vi "Select ROI Statistics Dialog.vi"(8 "error in (no error)":errorcluster) -> (0 "error out":errorcluster, 1 "OK?":bool caption="OK", 3 "ROI Statistics out":T1)   [LabVIEW 2021, in "Image.lvlib"]
doc: "Asks the user to select which ROI characteristics needs to be computed."
uses:
  Image.lvlib
  Image ROI Statistics Selection.ctl
panel:
  in  "ROI Statistics":T1
  in  "Deselect All":bool
  in  "Select All":bool
  in  "Cancel":bool
  in  "OK":bool caption="OK2"
  # "Select ROI Characteristics:"
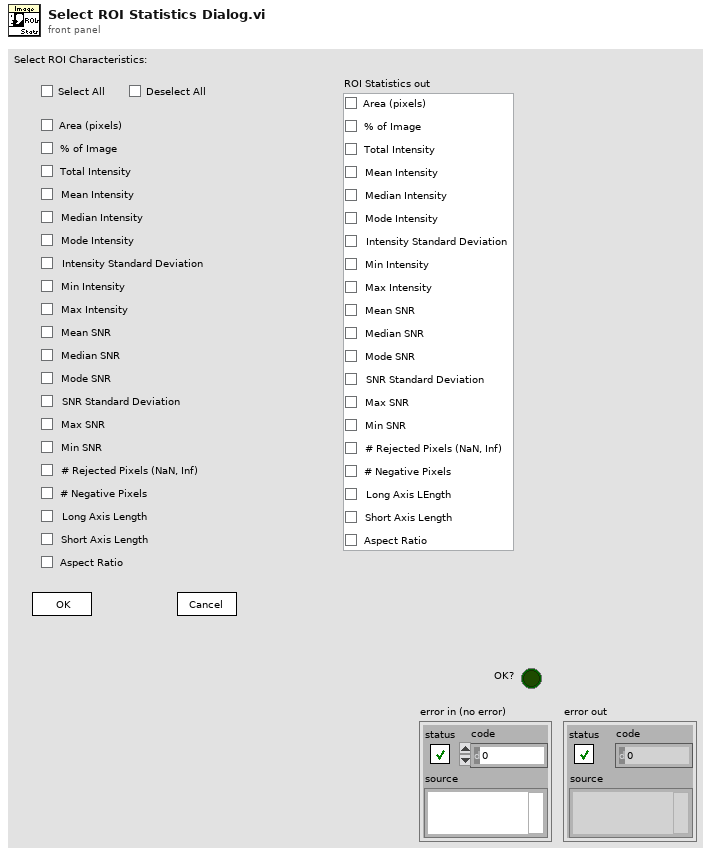
[diagram p1: front panel]
types:
  T1 = typedef "Image.lvlib/Image ROI Statistics Selection.ctl" = cluster{"Area (pixels)":bool, "% of Image":bool, "Total Intensity":bool, "Mean Intensity":bool, "Median Intensity":bool, "Mode Intensity":bool, "Intensity Standard Deviation":bool, "Min Intensity":bool, "Max Intensity":bool, "Mean SNR":bool, "Median SNR":bool, "Mode SNR":bool, "SNR Standard Deviation":bool, "Max SNR":bool, "Min SNR":bool, "# Rejected Pixels (NaN, Inf)":bool, "# Negative Pixels":bool, "Long Axis Length":bool, "Short Axis Length":bool, "Aspect Ratio":bool}
  T2 = enum32{"Invalid", "Standard", "Closed", "Hidden", "Minimized", "Maximized"}
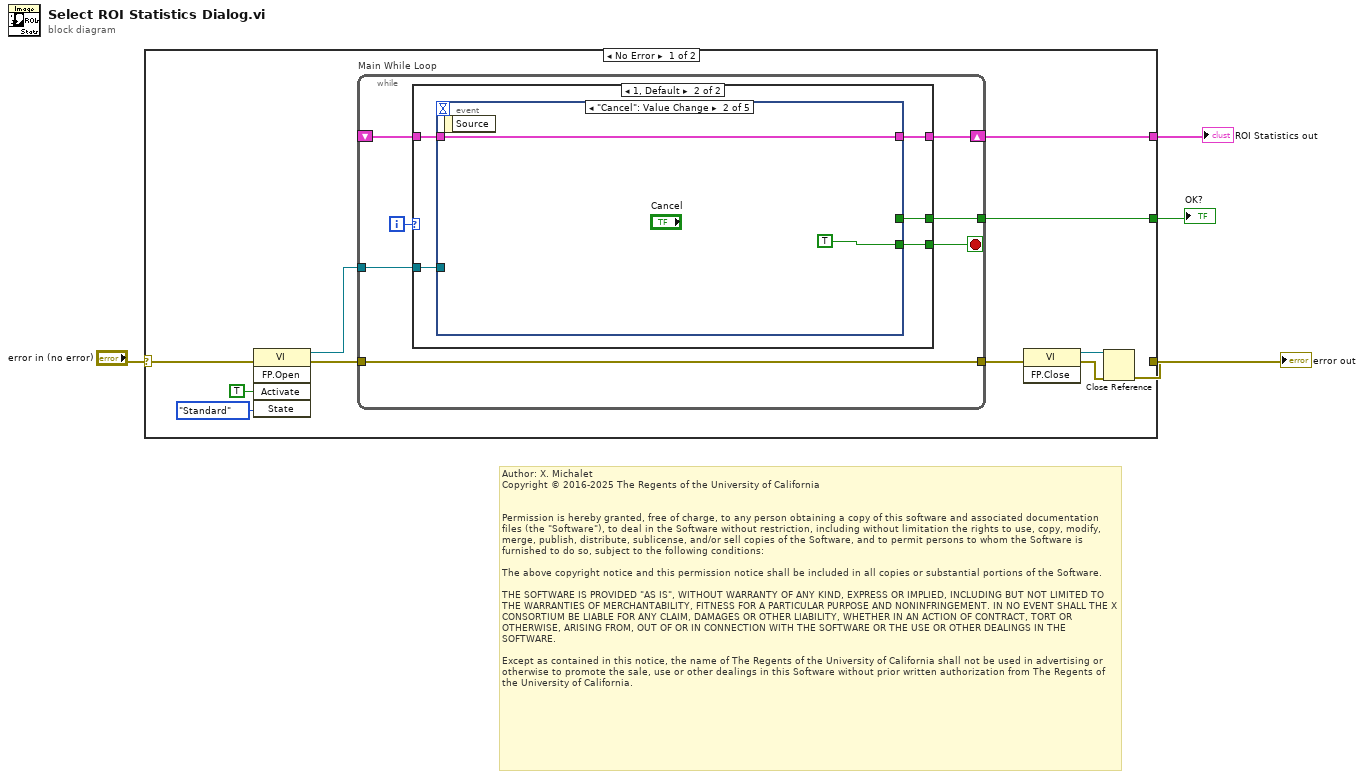
[diagram p0: block diagram]
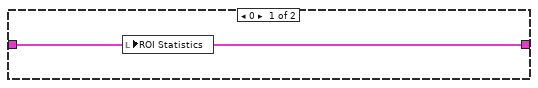
[diagram p2: hidden frame]
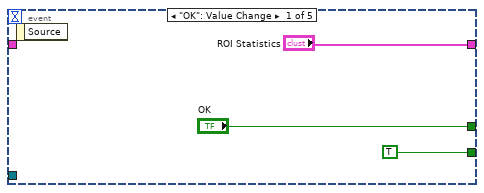
[diagram p3: hidden frame]
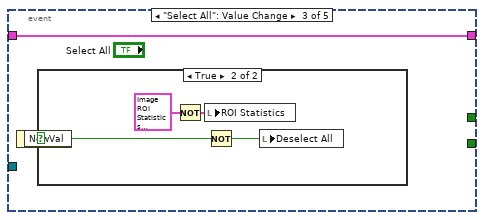
[diagram p4: hidden frame]
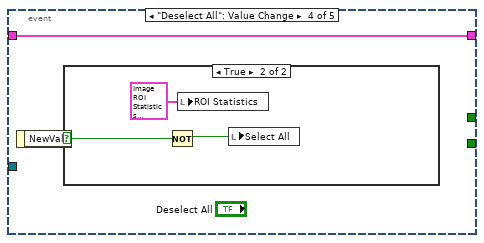
[diagram p6: hidden frame]
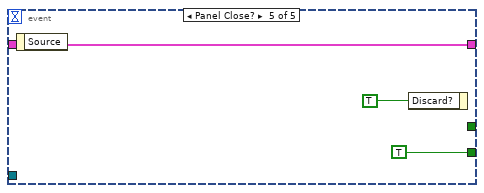
[diagram p8: hidden frame]
diagram:
  # "Author: X. Michalet\nCopyright © 2016-2025 The Regents of the University of California\n \n\nPermission is hereby granted, free of charge, to any person obtaining a copy of this software and associated documentation files (the \"Software\"), to deal in the Software without restriction, including without limitation the rights to use, copy, modify, merge, publish, distribute, sublicense, and/or sell copies of the Software, and to permit persons to whom the Software is furnished to do so, subject to the following conditions:\n\nThe above copyright notice and this permission notice shall be included in all copies or substantial portions of the Software.\n\nTHE SOFTWARE IS PROVIDED \"AS IS\", WITHOUT WARRANTY OF ANY KIND, EXPRESS OR IMPLIED, INCLUDING BUT NOT LIMITED TO THE WARRANTIES OF MERCHANTABILITY, FITNESS FOR A PARTICULAR PURPOSE AND NONINFRINGEMENT. IN NO EVENT SHALL THE X CONSORTIUM BE LIABLE FOR ANY CLAIM, DAMAGES OR OTHER LIABILITY, WHETHER IN AN ACTION OF CONTRACT, TORT OR OTHERWISE, ARISING FROM, OUT OF OR IN CONNECTION WITH THE SOFTWARE OR THE USE OR OTHER DEALINGS IN THE SOFTWARE.\n\nExcept as contained in this notice, the name of The Regents of the University of California shall not be used in advertising or otherwise to promote the sale, use or other dealings in this Software without prior written authorization from The Regents of the University of California."
  n1 = case shown="No Error" "error in (no error)" {
    selector: "error in (no error)" -> [w10 w48]
    tunnel: [w15 _] -> w4
    tunnel: [w9 w48] -> w2
    tunnel: [w8 _] -> w1
    frame No Error {
      n2 = invoke class="VI" method="FP.Open"(error in=w10, "Activate"=TRUE ("Activate?"), "State"=T2."Standard") -> (reference out=w5:refnum<vi>, error out=w7:errorcluster)  [unwired: 2 in, 3 out]
      n3 = while "Main While Loop" {
        tunnel: [w22] -> w15
        shift-right: [w19] -> w8
        shift-left: _ -> [w18]
        tunnel: w7 -> [w17]
        tunnel: [w17] -> w6
        tunnel: w5 -> [w16]
        i -> [w20]
        stop <- w21 stop-if-true
        n4 = case shown="1, Default" w20 {
          tunnel: [_ w28] -> w22
          tunnel: [_ w27] -> w21
          tunnel: [w23 w26] -> w19
          tunnel: w18 -> [w23 w25]
          tunnel: w16 -> [_ w24]
          frame 0 {
            n5 = local write "ROI Statistics"(w23) -> ()
          }
          frame 1, Default {
            n6 = event shown="[1] \"Cancel\": Value Change" {
              selector: _ -> [_ _ _ _ _]
              dyn-events: _ -> [_ _ _ _ _]
              timeout: _ -> [_ _ _ _ _]
              tunnel: ["OK" _ _ _ _] -> w28
              tunnel: [TRUE TRUE _ _ TRUE] -> w27
              tunnel: ["ROI Statistics" w32 w34 w40 w45] -> w26
              tunnel: w25 -> [_ w32 w34 w40 w45]
              tunnel: w24 -> [_ _ _ _ _]
              event "OK": Value Change {
                n7 = event-data() -> ()  [unwired: 1 in, 1 out]
              }
              event "Cancel": Value Change {
                n8 = event-data() -> ()  [unwired: 1 in, 1 out]
              }
              event "Select All": Value Change {
                n9 = event-data() -> ("NewVal"=w35:bool)  [unwired: 1 in]
                n10 = case shown="True" w35 {
                  selector: w35 -> [_ w39]
                  frame False {
                  }
                  frame True {
                    n11 = Not(x=T1 {"Area (pixels)"=FALSE, "% of Image"=FALSE, "Total Intensity"=FALSE, "Mean Intensity"=FALSE, "Median Intensity"=FALSE, "Mode Intensity"=FALSE, "Intensity Standard Deviation"=FALSE, "Min Intensity"=FALSE, "Max Intensity"=FALSE, "Mean SNR"=FALSE, "Median SNR"=FALSE, "Mode SNR"=FALSE, "SNR Standard Deviation"=FALSE, "Max SNR"=FALSE, "Min SNR"=FALSE, "# Rejected Pixels (NaN, Inf)"=FALSE, "# Negative Pixels"=FALSE, "Long Axis Length"=FALSE, "Short Axis Length"=FALSE, "Aspect Ratio"=FALSE} ("ROI Statistics")) -> (.not. x?=w36:T1)
                    n12 = local write "ROI Statistics"(w36) -> ()
                    n13 = Not(x=w39) -> (.not. x?=w38:bool)
                    n14 = local write "Deselect All"(w38) -> ()
                  }
                }
              }
              event "Deselect All": Value Change {
                n15 = event-data() -> ("NewVal"=w41:bool)  [unwired: 1 in]
                n16 = case shown="True" w41 {
                  selector: w41 -> [_ w44]
                  frame False {
                  }
                  frame True {
                    n17 = Not(x=w44) -> (.not. x?=w43:bool)
                    n18 = local write "ROI Statistics"(T1 {"Area (pixels)"=FALSE, "% of Image"=FALSE, "Total Intensity"=FALSE, "Mean Intensity"=FALSE, "Median Intensity"=FALSE, "Mode Intensity"=FALSE, "Intensity Standard Deviation"=FALSE, "Min Intensity"=FALSE, "Max Intensity"=FALSE, "Mean SNR"=FALSE, "Median SNR"=FALSE, "Mode SNR"=FALSE, "SNR Standard Deviation"=FALSE, "Max SNR"=FALSE, "Min SNR"=FALSE, "# Rejected Pixels (NaN, Inf)"=FALSE, "# Negative Pixels"=FALSE, "Long Axis Length"=FALSE, "Short Axis Length"=FALSE, "Aspect Ratio"=FALSE} ("ROI Statistics")) -> ()
                    n19 = local write "Select All"(w43) -> ()
                  }
                }
              }
              event Panel Close? {
                n20 = event-data() -> ()  [unwired: 1 in, 1 out]
                n21 = event-data("Discard?"=TRUE) -> ()  [unwired: 1 in, 1 out]
              }
            }
          }
        }
      }
      n22 = invoke class="VI" method="FP.Close"(error in=w6) -> (reference out=w12:refnum<vi>, error out=w11:errorcluster)  [unwired: 2 in, 1 out]
      n23 = Close Reference(reference=w12, error in (no error)=w11) -> (error out=w9:errorcluster)
    }
    frame Error {
    }
  }
  "OK?" <- w4
  "error out" <- w2
  "ROI Statistics out" <- w1
